vi "Read Server address.vi"(8 "error in (no error)":errorcluster, 11 "Red Pitaya Digitizer in":refnum<class "Red Pitaya Digitizer.lvclass">) -> (0 "error out":errorcluster, 2 "Server address":string="192.168.1.100", 3 "Red Pitaya Digitizer out":refnum<class "Red Pitaya Digitizer.lvclass">)   [LabVIEW 2015, in "Red Pitaya Digitizer.lvclass"]
uses:
  Red Pitaya Digitizer.lvclass
  Red Pitaya Digitizer.lvclass/Red Pitaya Digitizer.ctl
  RP Core/RP Instrument/RP Instrument.lvclass
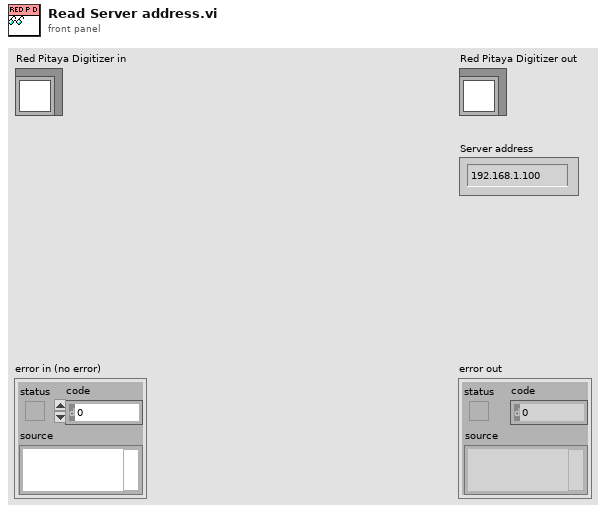
[diagram p1: front panel]
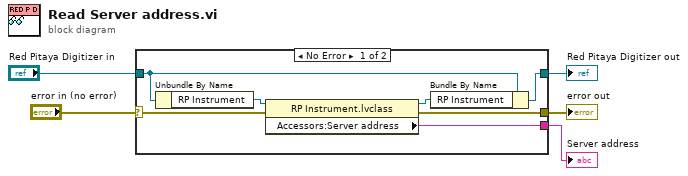
[diagram p0: block diagram]
diagram:
  n1 = case shown="No Error" "error in (no error)" {
    selector: "error in (no error)" -> [w7 w13]
    tunnel: [w6 w13] -> w4
    tunnel: [w9 w14] -> w2
    tunnel: "Red Pitaya Digitizer in" -> [w12 w14]
    tunnel: [w10 _] -> w1
    frame No Error {
      n2 = Unbundle By Name(w12) -> ("RP Instrument"=w11:refnum<class "RP Instrument.lvclass">)
      n3 = property class="RP Instrument.lvclass"(reference=w11, error in=w7) -> (reference out=w8:refnum<class "RP Instrument.lvclass">, error out=w6:errorcluster, "Accessors:Server address"=w10:string)
      n4 = Bundle By Name(cluster=w12, "RP Instrument"=w8) -> (w9:refnum<class "Red Pitaya Digitizer.lvclass">)
    }
    frame Error {
    }
  }
  "error out" <- w4
  "Red Pitaya Digitizer out" <- w2
  "Server address" <- w1
